vi "TCam_VerticalLines.vi"(7 "Width":u32, 8 "error in (no error)":errorcluster, 9 "Cluster":T1={"Core"={"Current VI Reference"=refnum, "Close Panel on Exit?"=FALSE}, "Image Out"=refnum, "State"=0, "Points"={"Top Left"={"X"=0.0, "Y"=0.0}, "Top Right"={"X"=0.0, "Y"=0.0}, "Bottom Left"={"X"=0.0, "Y"=0.0}, "Bottom Right"={"X"=0.0, "Y"=0.0}, "x space 2"=0.0, "y space 2"=0.0, "x_space"=0.0, "y_space"=0.0, "Pixels"=[], "Fixpoint"={"X"=0.0, "Y"=0.0}}, "img_array"=[], "Temps"=[], "Temps_Array"=[], "Scan Area"=0.0, "Fixpoint Area"=0.0, "Config"={"Freezing"={"Cutoff"=2.0, "EndIndex"=2}}, "PCR Size"=0, "ImageCount"=0, "ShowGradient"=FALSE, "Save Well data"=FALSE, "Save Blackbody data"=FALSE, "Save Temps For Offset"=FALSE} {"Points"."Bottom Right"."Y" format="%.2f"; "Points"."Bottom Right"."X" format="%.2f"; "Points"."Top Left"."Y" format="%.2f"; "Points"."Top Left"."X" format="%.2f"; "Points"."Top Right"."Y" format="%.2f"; "Points"."Top Right"."X" format="%.2f"; "Points"."Bottom Left"."Y" format="%.2f"; "Points"."Bottom Left"."X" format="%.2f"; "Points"."Fixpoint"."Y" format="%.2f"; "Points"."Fixpoint"."X" format="%.2f"}, 11 "Refnum in":T2) -> (0 "error out":errorcluster, 3 "Refnum out":T2)   [LabVIEW 2024]
uses:
  <vilib>/vision/Image Controls.llb/IMAQ Image.ctl
  DataCluster_TCAL.ctl
  TCE_Config.ctl
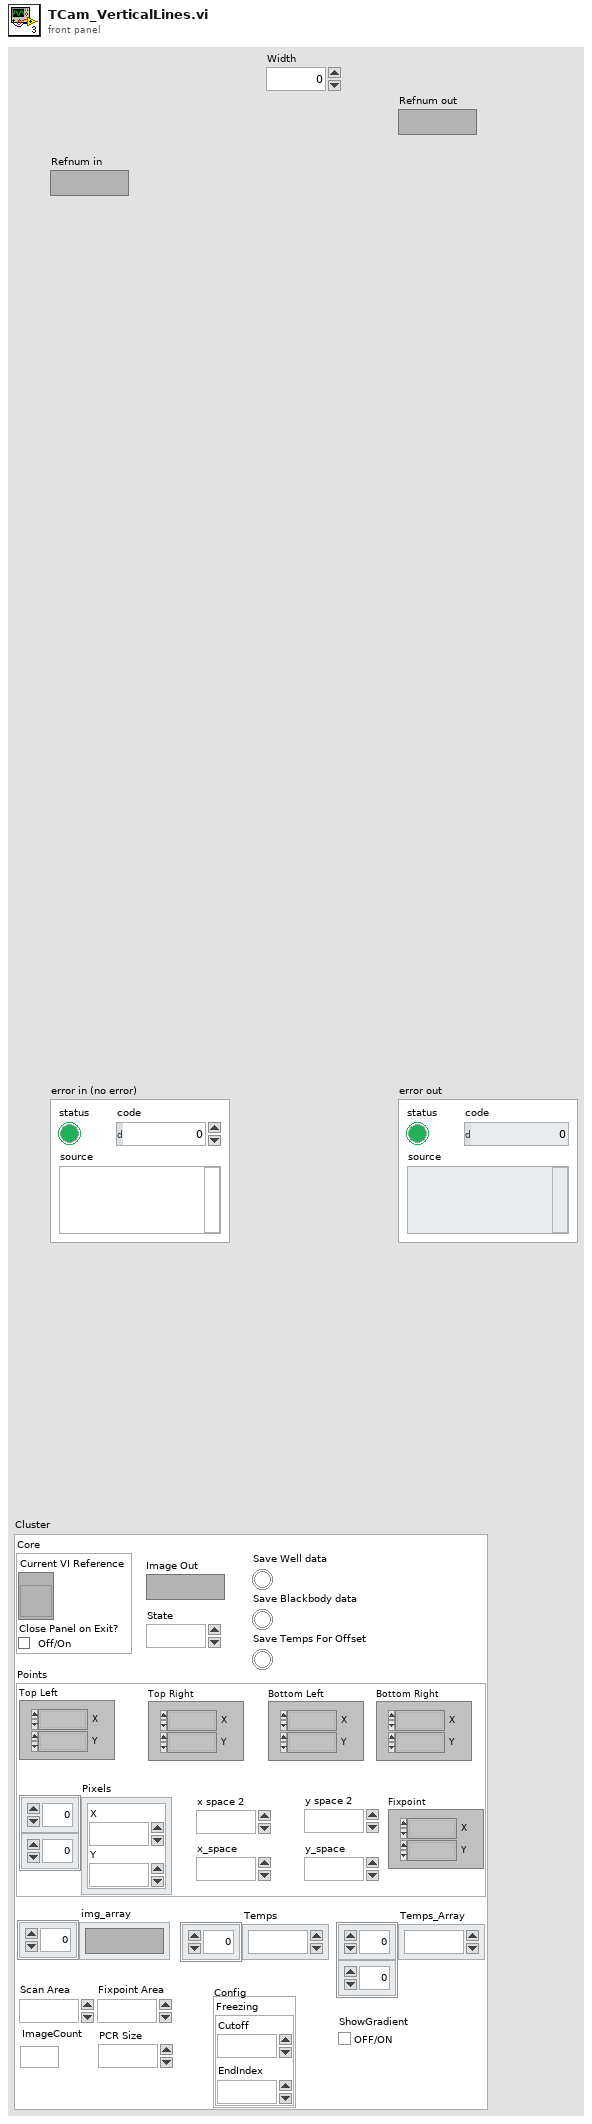
[diagram p1: front panel]
types:
  T1 = typedef "DataCluster_TCAL.ctl" = cluster{"Core":cluster{"Current VI Reference":refnum<vi>, "Close Panel on Exit?":bool}, "Image Out":T2, "State":i32, "Points":cluster{"Top Left":T3, "Top Right":T3, "Bottom Left":T3, "Bottom Right":T3, "x space 2":dbl, "y space 2":sgl, "x_space":sgl, "y_space":sgl, "Pixels":cluster{"X":i32, "Y":i32}[][], "Fixpoint":T3}, "img_array":T2[], "Temps":dbl[], "Temps_Array":dbl[][], "Scan Area":dbl, "Fixpoint Area":dbl, "Config":T4, "PCR Size":u16, "ImageCount":i32, "ShowGradient":bool, "Save Well data":bool, "Save Blackbody data":bool, "Save Temps For Offset":bool}
  T2 = typedef "IMAQ Image.ctl" = refnum<image>
  T3 = typedef "IMAQ Point" = cluster{"X":sgl, "Y":sgl}
  T4 = typedef "TCE_Config.ctl" = cluster{"Freezing":cluster{"Cutoff":dbl, "EndIndex":i32}}
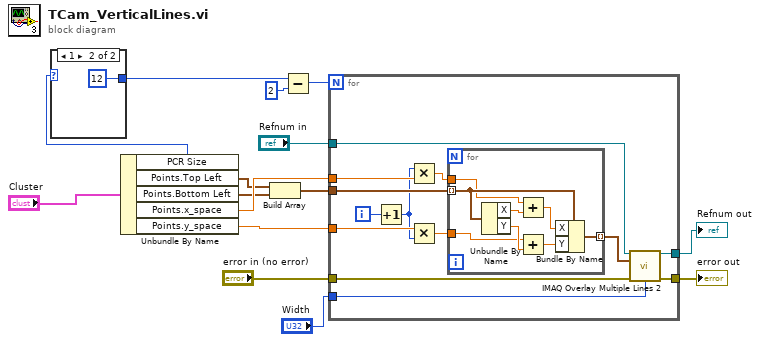
[diagram p0: block diagram]
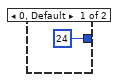
[diagram p2: hidden frame]
diagram:
  n1 = Unbundle By Name("Cluster") -> ("PCR Size"=w1:u16, "Points.Top Left"=w8:T3, "Points.Bottom Left"=w9:T3, "Points.x_space"=w12:sgl, "Points.y_space"=w11:sgl)
  n2 = case shown="1" w1 {
    tunnel: [24 12] -> w15
    frame 0, Default {
    }
    frame 1 {
    }
  }
  n3 = Build Array(w8, w9) -> (w10:T3[])
  n4 = Subtract(x=w15, y=u16 2) -> (x-y=w13:i32)
  n5 = for {
    N: w13 -> [_]
    tunnel: "Refnum in" -> [w30]
    tunnel: [w29] -> w4
    tunnel: "error in (no error)" -> [w28]
    tunnel: [w27] -> w6
    tunnel: "Width" -> [w26]
    tunnel: w10 -> [w25]
    tunnel: w11 -> [w24]
    tunnel: w12 -> [w23]
    i -> [w20]
    n6 = Increment(x=w20) -> (x+1=w18:i32)
    n7 = Multiply(x=w18, y=w23) -> (x*y=w19:sgl)
    n8 = Multiply(x=w24, y=w18) -> (x*y=w21:sgl)
    n9 = for {
      tunnel: w25 -> [w38] mode=indexing
      tunnel: w21 -> [w33]
      tunnel: w19 -> [w32]
      tunnel: [w31] -> w22 mode=indexing
      n10 = Unbundle By Name(w38) -> ("X"=w37:sgl, "Y"=w35:sgl)
      n11 = Add(x=w32, y=w37) -> (x+y=w36:sgl)
      n12 = Add(x=w33, y=w35) -> (x+y=w34:sgl)
      n13 = Bundle By Name(cluster=w38, "X"=w36, "Y"=w34) -> (w31:T3)
    }
    n14 = call "IMAQ Overlay Multiple Lines 2"("Image"=w30, "Line End Points"=w22, "error in (no error)"=w28, "Width"=w26) -> ("Image Out"=w29:T2, "error out"=w27:errorcluster)  [unwired: 10 in]
  }
  "error out" <- w6
  "Refnum out" <- w4
